vi "Numeric EQ.vi"(11 "Data In":i32) -> (3 "Data Out":i32)   [LabVIEW 2018]
uses:
  Core/Assert API Components/Failure Actions.ctl
  Core/Assert API Components/Assert API Components.lvlib
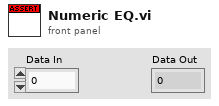
[diagram p1: front panel]
types:
  T1 = typedef "Assert API Components.lvlib/Failure Actions.ctl" = enum16{"None", "Log To File", "Pause Execution", "Abort Execution"}
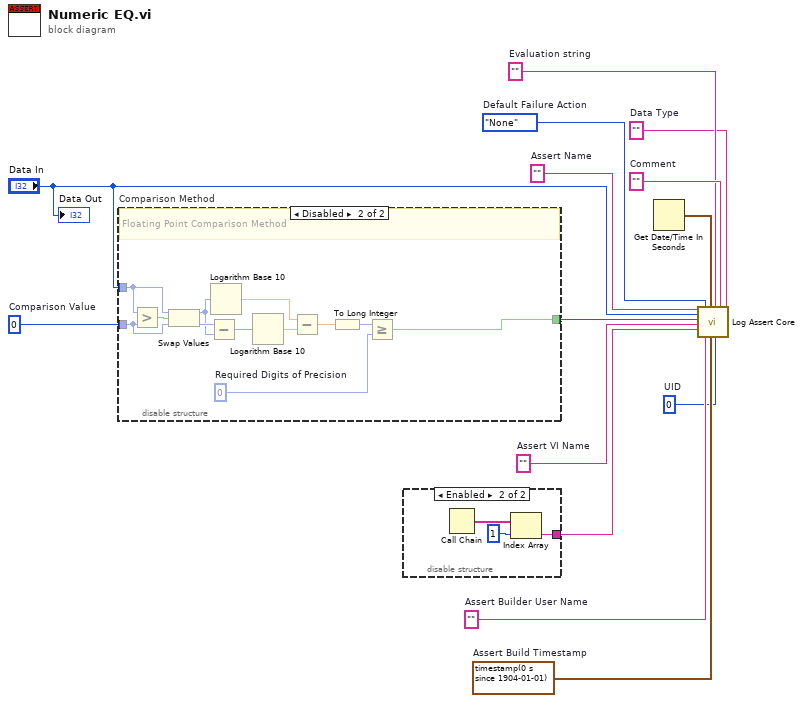
[diagram p0: block diagram]
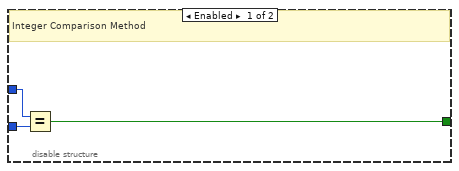
[diagram p2: hidden frame]
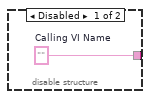
[diagram p3: hidden frame]
diagram:
  w2 = 0  # UID
  w4 = ""  # Assert VI Name
  w5 = timestamp(0 s since 1904-01-01)  # Assert Build Timestamp
  w6 = ""  # Assert Builder User Name
  w7 = ""  # Data Type
  w11 = ""  # Comment
  w8 = ""  # Evaluation string
  w13 = Failure_Actions."None"  # Default Failure Action
  w14 = ""  # Assert Name
  w12 = 0  # Comparison Value
  n1 = disable-structure "Comparison Method" shown="Disabled" {
    disable-tunnel: w12 -> [w17 w19]
    disable-tunnel: "Data In" -> [w16 w20]
    disable-tunnel: [w15 w18] -> w9
    frame Enabled {
      # "Integer Comparison Method"
      n2 = Equal?(x=w16, y=w17) -> (x = y?=w15:bool)
    }
    frame Disabled {
      w26 = 0  # Required Digits of Precision
      # "Floating Point Comparison Method"
      n3 = Greater?(x=w20, y=w19) -> (0:w27:bool)
      n4 = Swap Values(12:w20, 13:w27, 14:w19) -> (1:w28:i32, 3:w29:i32)
      n5 = Subtract(x=w29, y=w28) -> (x-y=w21:i32)
      n6 = Logarithm Base 10(1:w28) -> (0:w22:dbl)
      n7 = Logarithm Base 10(1:w21) -> (0:w23:dbl)
      n8 = Subtract(x=w22, y=w23) -> (x-y=w24:dbl)
      n9 = To Long Integer(number=w24) -> (32bit integer=w25:i32)
      n10 = Greater Or Equal?(x=w25, y=w26) -> (x >= y?=w18:bool)
    }
  }
  n11 = disable-structure shown="Enabled" {
    disable-tunnel: [w30 w31] -> w1
    frame Disabled {
      w30 = ""  # Calling VI Name
    }
    frame Enabled {
      n12 = Call Chain() -> (call chain=w32:string[])
      n13 = Index Array(array=w32, index=1) -> (element=w31:string)
    }
  }
  n14 = Get Date/Time In Seconds() -> (seconds since 1Jan1904=w3:timestamp)
  n15 = call "Log Assert Core.vi"("Assert Name"=w14, "Data Value"="Data In", "Status"=w9, "Assert VI Name"=w4, "Calling VI Name"=w1, "Failure Action"=w13, "Assert Builder User Name"=w6, "Last Update"=w3, "Assert Build Timestamp"=w5, "Evaluation String"=w8, "Assert VI UID"=w2, "Comment"=w11, "Data Type"=w7) -> ()  [unwired: 7 in]
  "Data Out" <- "Data In"
